vi "burn_warn_subVI.vi"(11 "Placeholder\nSfc Temp":dbl) -> (2 "Level":dbl, 3 "String":string)   [LabVIEW 2021]
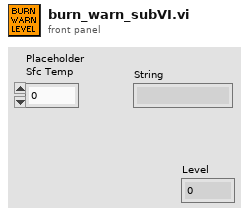
[diagram p1: front panel]
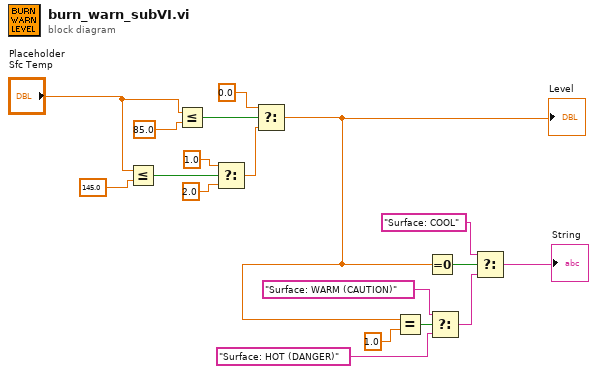
[diagram p0: block diagram]
diagram:
  n1 = Less Or Equal?(x="Placeholder\nSfc Temp", y=145.0) -> (x <= y?=w12:bool)
  n2 = Less Or Equal?(x="Placeholder\nSfc Temp", y=85.0) -> (x <= y?=w17:bool)
  n3 = Select(t=1.0, s=w12, f=2.0) -> (s? t:f=w10:dbl)
  n4 = Select(t=0.0, s=w17, f=w10) -> (s? t:f=w5:dbl)
  "Level" <- w5
  n5 = Equal?(x=w5, y=1.0) -> (x = y?=w4:bool)
  n6 = Equal To 0?(x=w5) -> (x = 0?=w9:bool)
  n7 = Select(t="Surface: WARM (CAUTION)", s=w4, f="Surface: HOT (DANGER)") -> (s? t:f=w1:string)
  n8 = Select(t="Surface: COOL", s=w9, f=w1) -> (s? t:f=→"String":string)
